vi "parse load report.vi"(8 "error in":errorcluster, 11 "message data":string) -> (0 "error out":errorcluster, 2 "load error":errorcluster, 3 "engine loaded":string)   [LabVIEW 2013, in "module execution process.lvlib"]
uses:
  module execution process.lvlib
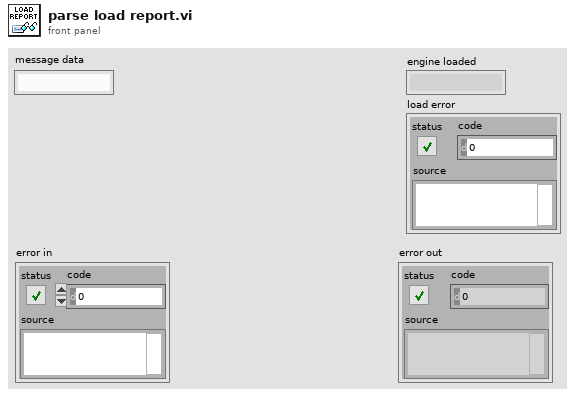
[diagram p1: front panel]
types:
  T1 = cluster{"engine loaded":string, "load error":errorcluster}
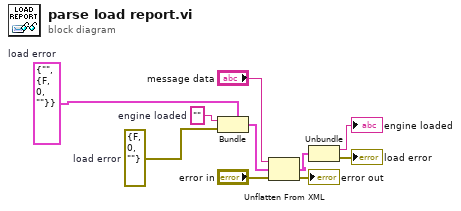
[diagram p0: block diagram]
diagram:
  w6 = T1 {"engine loaded"="", "load error"={"status"=FALSE, "code"=0, "source"=""}}  # load error
  w9 = errorcluster {"status"=FALSE, "code"=0, "source"=""}  # load error
  w10 = ""  # engine loaded
  n1 = Bundle(cluster=w6, "engine loaded"=w10, "load error"=w9) -> (w4:T1)
  n2 = Unflatten From XML(xml string="message data", type=w4, error in (no error)="error in") -> (value=w2:T1, error out=→"error out":errorcluster)
  n3 = Unbundle(w2) -> ("engine loaded"=→"engine loaded":string, "load error"=→"load error":errorcluster)
